vi "Set View Status.vi"(8 "error in (no error)":errorcluster, 9 "View Status":T1, 10 "View":string, 11 "GUI Container Actor in":refnum<class "GUI Container Actor.lvclass">) -> (0 "error out":errorcluster, 2 "Status Added":bool, 3 "GUI Container Actor out":refnum<class "GUI Container Actor.lvclass">)   [LabVIEW 2017, in "GUI Views.lvlib" / "GUI Container Actor.lvclass"]
uses:
  GUI Container Actor.lvclass
  typedefs/View Status.ctl
  <vilib>/ActorFramework/Message Enqueuer/Message Enqueuer.lvclass
  typedefs/View Details.ctl
  typedefs/FP Status.ctl
  GUI Container Actor.lvclass/GUI Container Actor.ctl
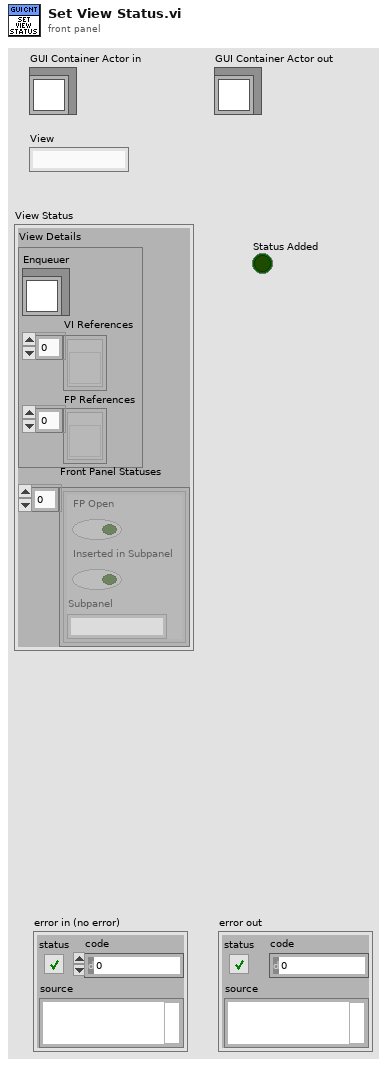
[diagram p1: front panel]
types:
  T1 = typedef "GUI Views.lvlib/GUI Container Actor.lvclass/View Status.ctl" = cluster{"View Details":T2, "Front Panel Statuses":T3[]}
  T2 = typedef "GUI Views.lvlib/GUI Container Actor.lvclass/View Details.ctl" = cluster{"Enqueuer":refnum<class "Message Enqueuer.lvclass">, "VI References":refnum<vi>[], "FP References":refnum<vi>[]}
  T3 = typedef "GUI Views.lvlib/GUI Container Actor.lvclass/FP Status.ctl" = cluster{"FP Open":bool, "Inserted in Subpanel":bool, "Subpanel":string}
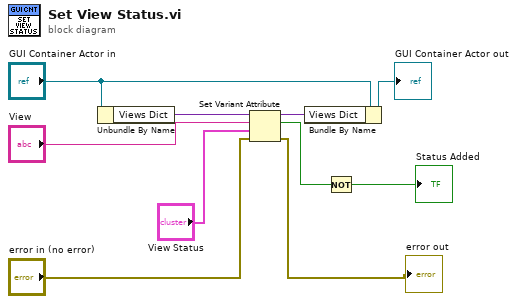
[diagram p0: block diagram]
diagram:
  n1 = Unbundle By Name("GUI Container Actor in") -> ("Views Dict"=w4:variant)
  n2 = Set Variant Attribute(Variant=w4, name="View", value="View Status", error in="error in (no error)") -> (Variant out=w7:variant, replaced=w2:bool, error out=→"error out":errorcluster)
  n3 = Bundle By Name(cluster="GUI Container Actor in", "Views Dict"=w7) -> (→"GUI Container Actor out":refnum<class "GUI Container Actor.lvclass">)
  n4 = Not(x=w2) -> (.not. x?=→"Status Added":bool)
